vi "Sort-To-XYZ.vi"(9 "位置 2":i32, 11 "位置":i32) -> (1 "輸出位移距離2":dbl[](array[numeric]), 3 "輸出移動距離":dbl[](array[numeric]), 5 "執行補值、校正?":bool)   [LabVIEW 2019]
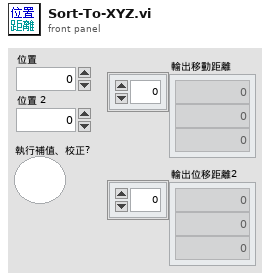
[diagram p1: front panel]
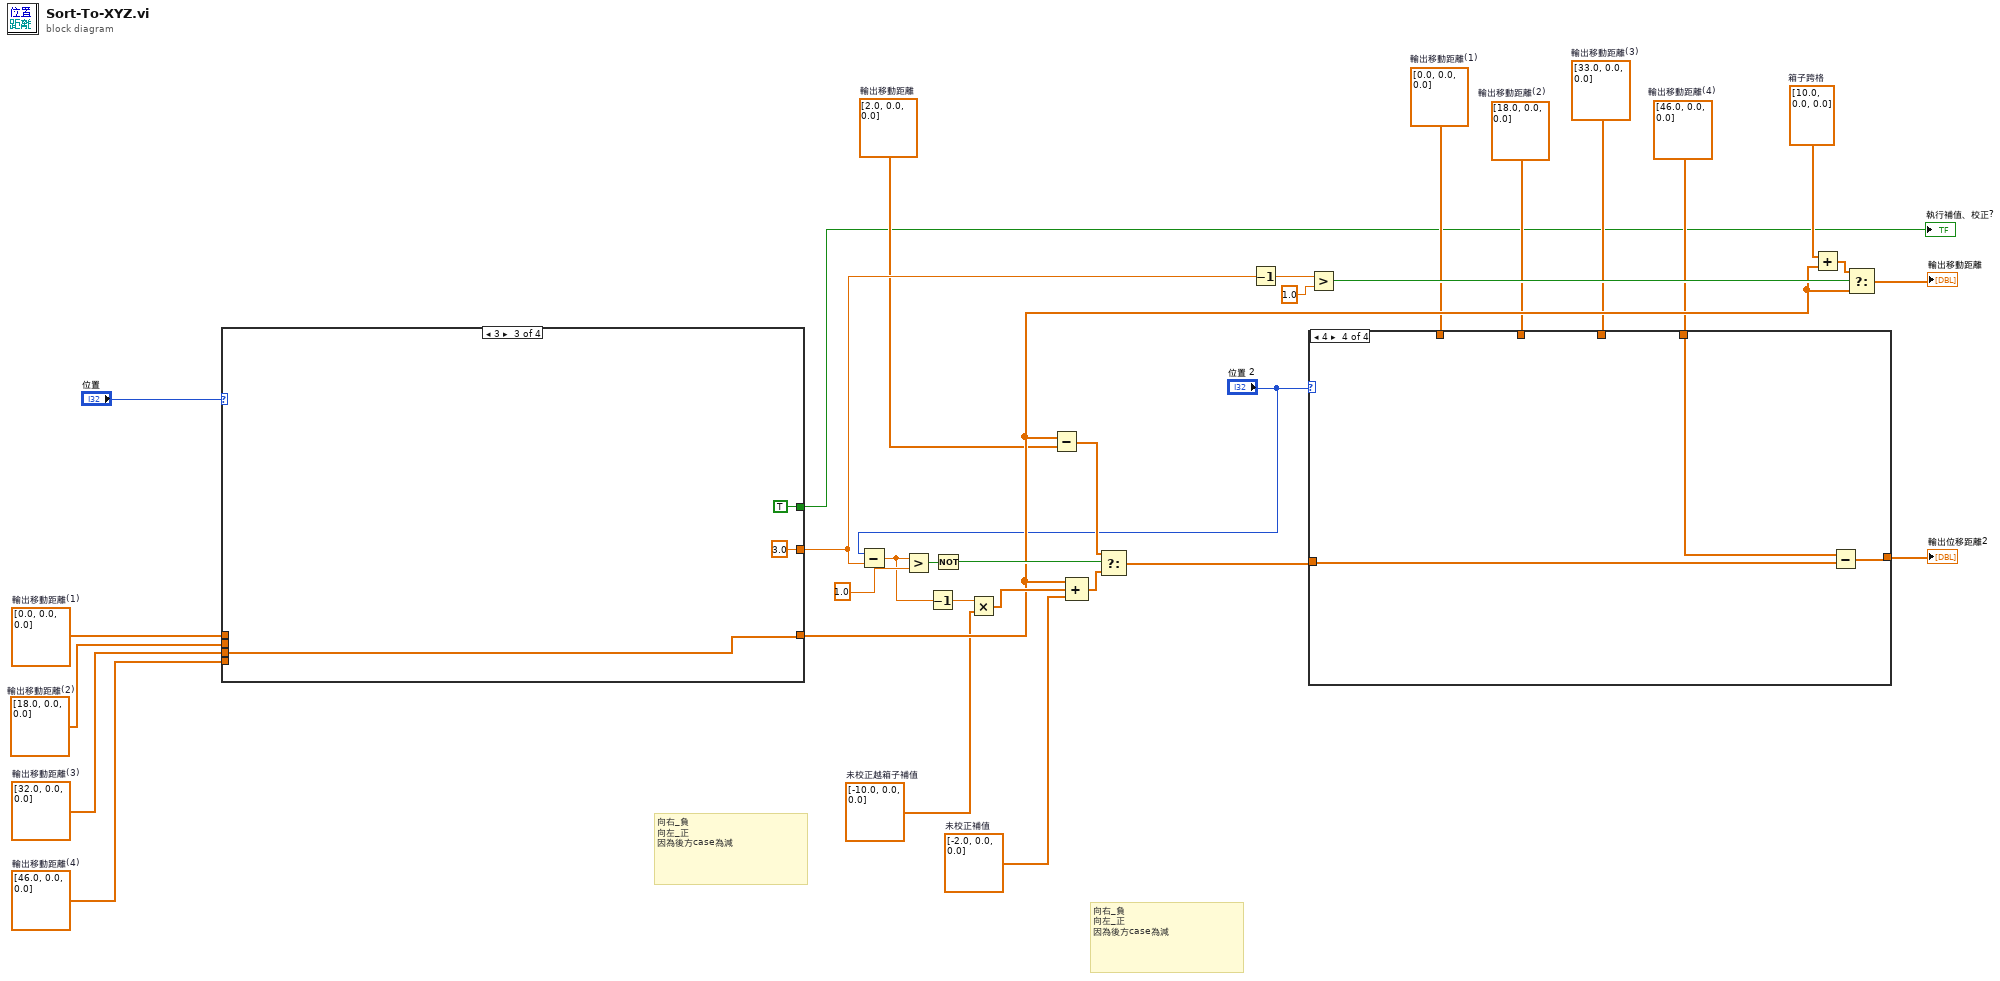
[diagram p0: block diagram]
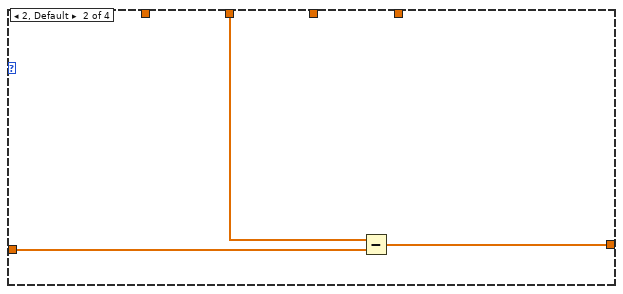
[diagram p3: hidden frame]
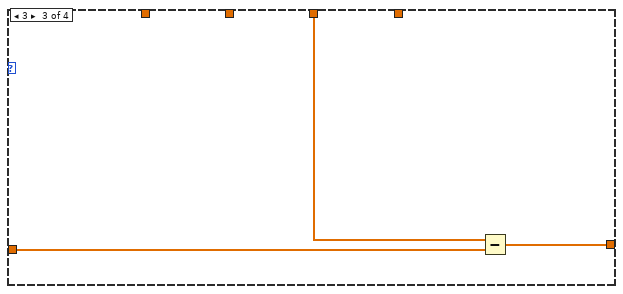
[diagram p4: hidden frame]
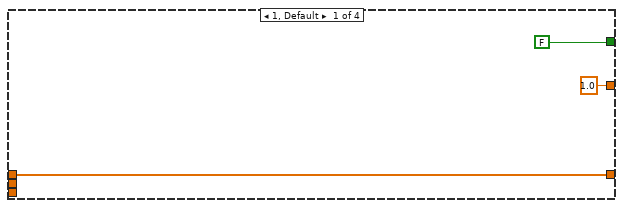
[diagram p5: hidden frame]
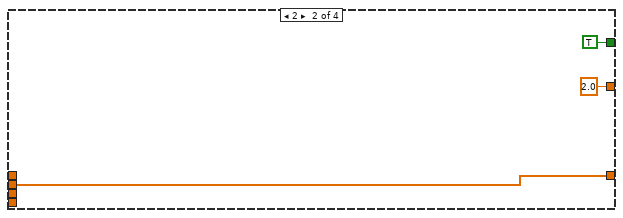
[diagram p6: hidden frame]
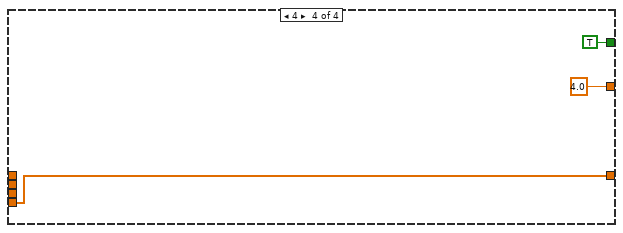
[diagram p7: hidden frame]
diagram:
  w7 = dbl[] [46.0, 0.0, 0.0]  # 輸出移動距離(4)
  w8 = dbl[] [33.0, 0.0, 0.0]  # 輸出移動距離(3)
  w9 = dbl[] [18.0, 0.0, 0.0]  # 輸出移動距離(2)
  w10 = dbl[] [0.0, 0.0, 0.0]  # 輸出移動距離(1)
  w5 = dbl[] [2.0, 0.0, 0.0]  # 輸出移動距離
  w6 = dbl[] [10.0, 0.0, 0.0]  # 箱子跨格
  w12 = dbl[] [46.0, 0.0, 0.0]  # 輸出移動距離(4)
  w13 = dbl[] [32.0, 0.0, 0.0]  # 輸出移動距離(3)
  w14 = dbl[] [18.0, 0.0, 0.0]  # 輸出移動距離(2)
  w15 = dbl[] [0.0, 0.0, 0.0]  # 輸出移動距離(1)
  w16 = dbl[] [-10.0, 0.0, 0.0]  # 未校正越箱子補值
  w17 = dbl[] [-2.0, 0.0, 0.0]  # 未校正補值
  # "向右_負\n向左_正\n因為後方case為減"
  # "向右_負\n向左_正\n因為後方case為減"
  n1 = case shown="3" "位置" {
    tunnel: [w33 w36 w39 w42] -> w20
    tunnel: [FALSE TRUE TRUE TRUE] -> w4
    tunnel: [1.0 2.0 3.0 4.0] -> w18
    tunnel: w15 -> [w33 _ _ _]
    tunnel: w14 -> [_ w36 _ _]
    tunnel: w13 -> [_ _ w39 _]
    tunnel: w12 -> [_ _ _ w42]
    frame 1, Default {
    }
    frame 2 {
    }
    frame 3 {
    }
    frame 4 {
    }
  }
  "執行補值、校正?" <- w4
  n2 = Subtract(x="位置 2", y=w18) -> (x-y=w26:dbl)
  n3 = Greater?(x=w26, y=1.0) -> (0:w25:bool)
  n4 = Decrement(x=w26) -> (x-1=w27:dbl)
  n5 = Not(x=w25) -> (.not. x?=w24:bool)
  n6 = Multiply(x=w27, y=w16) -> (x*y=w29:dbl[])
  n7 = Subtract(x=w20, y=w5) -> (x-y=w28:dbl[])
  n8 = Compound Arithmetic op=ADD(w20, w29, w17) -> (w32:dbl[])
  n9 = Select(t=w28, s=w24, f=w32) -> (s? t:f=w31:dbl[])
  n10 = Decrement(x=w18) -> (x-1=w19:dbl)
  n11 = Greater?(x=w19, y=1.0) -> (0:w22:bool)
  n12 = case shown="4" "位置 2" {
    tunnel: w31 -> [_ w48 w51 w54]
    tunnel: [w45 w47 w50 w53] -> w2
    tunnel: w10 -> [w45 _ _ _]
    tunnel: w9 -> [_ w46 _ _]
    tunnel: w8 -> [_ _ w49 _]
    tunnel: w7 -> [_ _ _ w52]
    frame 1 {
    }
    frame 2, Default {
      n13 = Subtract(x=w46, y=w48) -> (x-y=w47:dbl[])
    }
    frame 3 {
      n14 = Subtract(x=w49, y=w51) -> (x-y=w50:dbl[])
    }
    frame 4 {
      n15 = Subtract(x=w52, y=w54) -> (x-y=w53:dbl[])
    }
  }
  "輸出位移距離2" <- w2
  n16 = Add(x=w6, y=w20) -> (x+y=w21:dbl[])
  n17 = Select(t=w21, s=w22, f=w20) -> (s? t:f=→"輸出移動距離":dbl[])
